vi "scale kalman input.vi"(6 "t scale factor":dbl=2.5e-08, 7 "x scale factors":dbl[](array[numeric])=[0.016, 0.016, 0.00025], 10 "kalman result":T2) -> (2 "kalman result scaled":T1)   [LabVIEW 2010]
uses:
  kalman_result_unscaled.ctl
  kalman_result_scaled.ctl
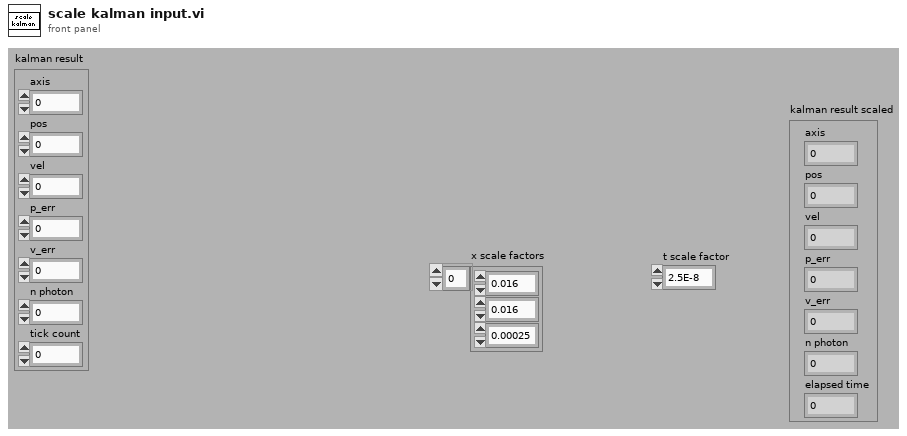
[diagram p1: front panel]
types:
  T1 = typedef "kalman_result_scaled.ctl" = cluster{"axis":u8, "pos":dbl, "vel":dbl, "p_err":dbl, "v_err":dbl, "n photon":u32, "elapsed time":dbl}
  T2 = typedef "kalman_result_unscaled.ctl" = cluster{"axis":u8, "pos":i16, "vel":i16, "p_err":i16, "v_err":i16, "n photon":u32, "tick count":u32}
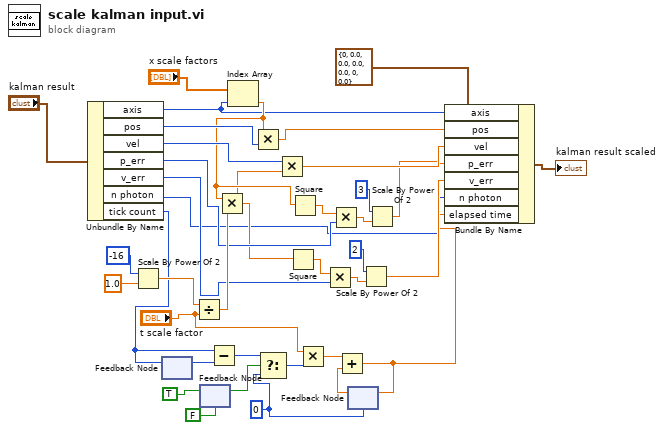
[diagram p0: block diagram]
diagram:
  w10 = 0
  n1 = Unbundle By Name("kalman result") -> ("axis"=w8:u8, "pos"=w36:i16, "vel"=w35:i16, "p_err"=w28:i16, "v_err"=w21:i16, "n photon"=w3:u32, "tick count"=w19:u32)
  n2 = Scale By Power Of 2(n=-16, x=1.0) -> (x*2^n=w32:dbl)
  n3 = feedback-in #1(w19) -> ()
  n4 = feedback #1() -> (w20:u32)  [unwired: 1 in]
  n5 = Divide(x=w32, y="t scale factor") -> (x/y=w31:dbl)
  n6 = feedback-in #2(TRUE ("s")) -> ()
  n7 = feedback #2(FALSE ("s")) -> (w15:bool)
  n8 = Subtract(x=w19, y=w20) -> (x-y=w18:u32)
  n9 = Index Array(array="x scale factors", index=w8) -> (element=w30:dbl)
  n10 = Multiply(x=w30, y=w31) -> (x*y=w25:dbl)
  n11 = Multiply(x=w30, y=w36) -> (x*y=w7:dbl)
  n12 = Select(t=w18, s=w15, f=w10) -> (s? t:f=w14:u32)
  n13 = Multiply(x=w35, y=w25) -> (x*y=w6:dbl)
  n14 = Square(x=w25) -> (x^2=w22:dbl)
  n15 = Square(x=w30) -> (x^2=w29:dbl)
  n16 = Multiply(x="t scale factor", y=w14) -> (x*y=w12:dbl)
  n17 = Multiply(x=w22, y=w21) -> (x*y=w24:dbl)
  n18 = Multiply(x=w29, y=w28) -> (x*y=w27:dbl)
  n19 = feedback #3(w10) -> (w11:dbl)
  n20 = Add(x=w12, y=w11) -> (x+y=w2:dbl)
  n21 = feedback-in #3(w2) -> ()
  n22 = Scale By Power Of 2(n=2, x=w24) -> (x*2^n=w4:dbl)
  n23 = Scale By Power Of 2(n=3, x=w27) -> (x*2^n=w5:dbl)
  n24 = Bundle By Name(cluster=T1 {"axis"=0, "pos"=0.0, "vel"=0.0, "p_err"=0.0, "v_err"=0.0, "n photon"=0, "elapsed time"=0.0} ("kalman result scaled"), "axis"=w8, "pos"=w7, "vel"=w6, "p_err"=w5, "v_err"=w4, "n photon"=w3, "elapsed time"=w2) -> (→"kalman result scaled":T1)
